vi "AssetInterface_Write Asset.vi"(8 "error in (no error)":errorcluster, 10 "TagBus DVR":refnum<data-value>, 11 "Asset_Interface in":refnum<class "Load.lvclass">) -> (0 "error out":errorcluster, 2 "TagBus DVR out":refnum<data-value>, 3 "Asset_Interface out":refnum<class "Load.lvclass">)   [LabVIEW 2015, in "Load.lvclass"]
uses:
  Load.lvclass
  TagBus/TagBus.lvclass
  AssetInterface.lvclass
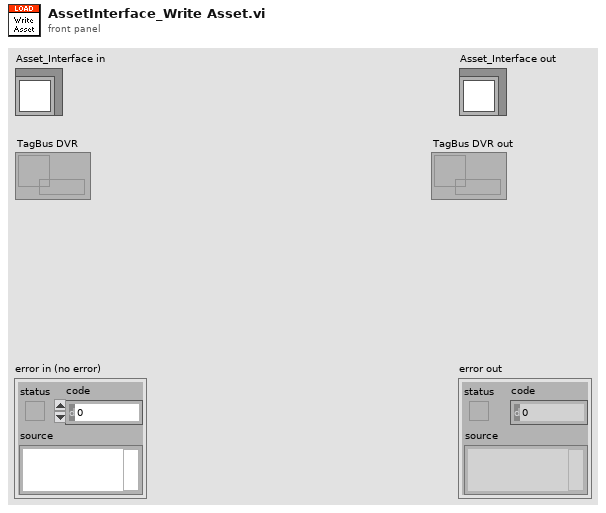
[diagram p1: front panel]
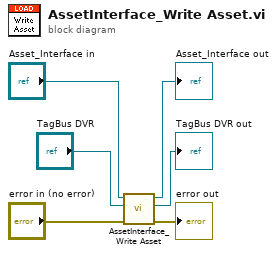
[diagram p0: block diagram]
diagram:
  n1 = call-parent "AssetInterface_Write Asset.vi"("error in (no error)"="error in (no error)", "TagBus DVR"="TagBus DVR", "Asset_Interface in"="Asset_Interface in") -> ("error out"=→"error out":errorcluster, "TagBus DVR out"=→"TagBus DVR out":refnum<data-value>, "Asset_Interface out"=→"Asset_Interface out":refnum<class "Load.lvclass">)  [unwired: 6 in]
